vi ".NET Process Tester.vi"() -> ()   [LabVIEW 2019]
uses:
  .NET Process/.NET Process.lvclass
panel:
  out "ErrOut":string
  out "StdOut":string
  in  "Send":bool
  in  "Cmd In":string
  in  "Stop":bool
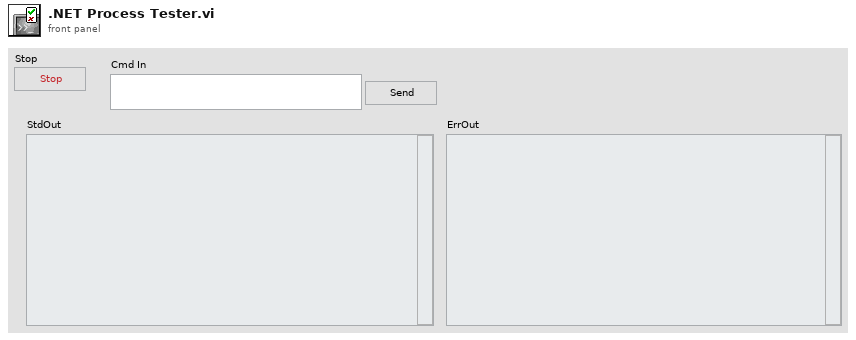
[diagram p1: front panel]
types:
  T1 = cluster{"StdOut Event":refnum<user-event>, "StdErr Event":refnum<user-event>}
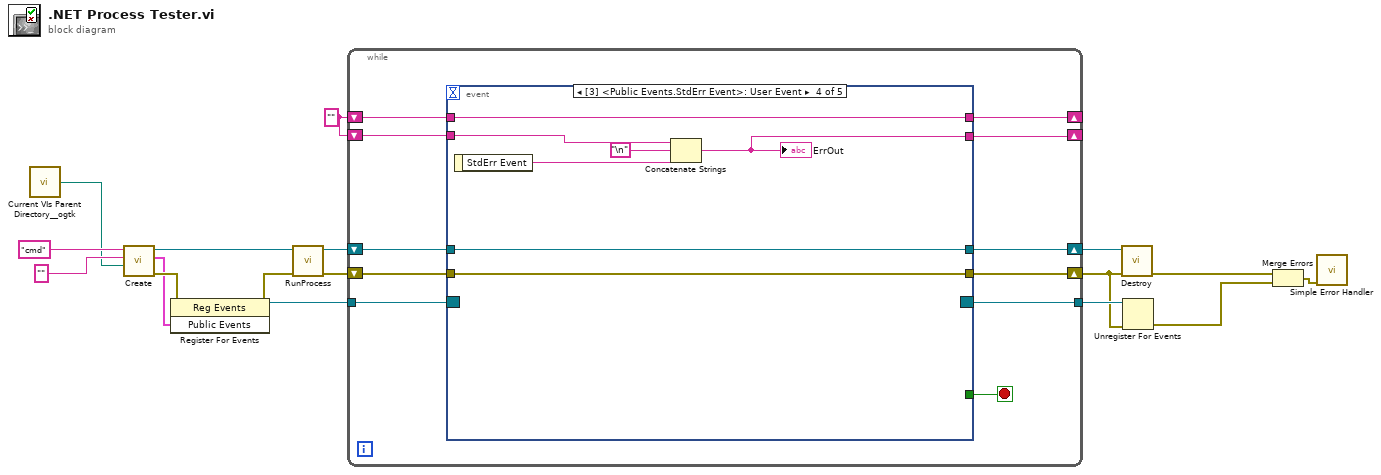
[diagram p0: block diagram]
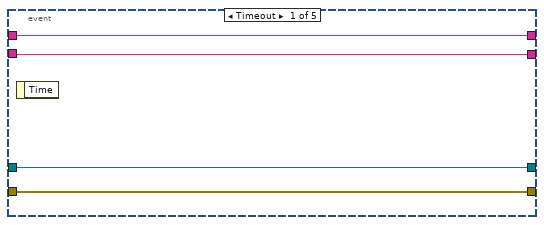
[diagram p2: hidden frame]
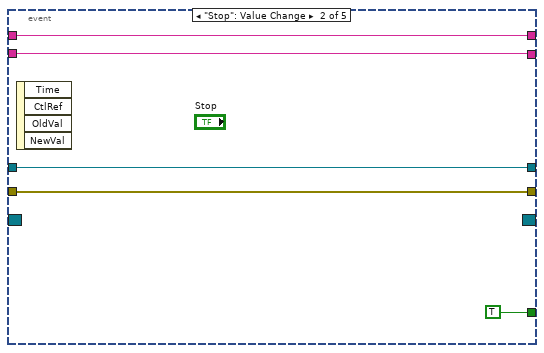
[diagram p3: hidden frame]
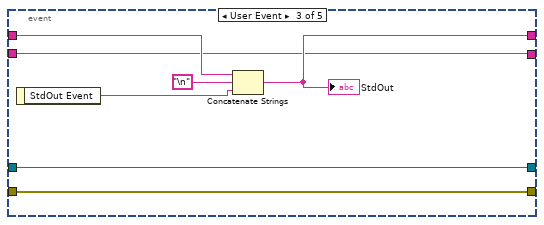
[diagram p4: hidden frame]
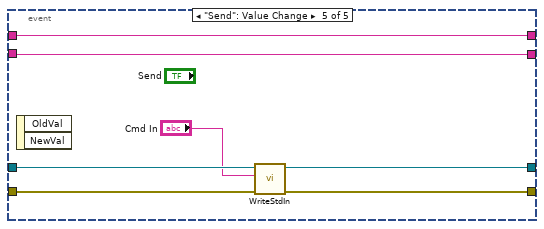
[diagram p5: hidden frame]
diagram:
  w7 = ""
  n1 = call "Current VIs Parent Directory__ogtk.vi"() -> ("Parent Directory (+ Relative)"=w5:path)  [unwired: 5 in]
  n2 = call "Create.vi"("Working Directory (App Directory)"=w5, "Arguments (empty)"="" ("Process File Name"), "Process File Name"="cmd") -> ("error out"=w3:errorcluster, "Public Events"=w1:T1, ".NET Process out"=w15:refnum<class ".NET Process.lvclass">)  [unwired: 6 in]
  n3 = register-events(error in=w3, w1) -> (reference out=w14:refnum<event-registration>, error out=w2:errorcluster)  [unwired: 1 in]
  n4 = call "RunProcess.vi"("error in (no error)"=w2, ".NET Process in"=w15) -> ("error out"=w4:errorcluster, ".NET Process out"=w17:refnum<class ".NET Process.lvclass">)  [unwired: 8 in]
  n5 = while {
    shift-right: [w28] -> w16
    shift-left: w17 -> [w27]
    shift-right: [w25] -> w12
    shift-left: w4 -> [w26]
    tunnel: w14 -> [w24]
    tunnel: [w23] -> w13
    shift-right: [w21] -> _
    shift-left: w7 -> [w22]
    shift-right: [w18] -> _
    shift-left: w7 -> [w19]
    stop <- w20 stop-if-true
    n6 = event shown="[3] <Public Events.StdErr Event>: User Event" {
      selector: w24 -> [_ _ _ _ _]
      dyn-events: [_ _ _ _ _] -> w23
      timeout: _ -> [_ _ _ _ _]
      tunnel: [w32 w37 w44 w51 w58] -> w28
      tunnel: w27 -> [w32 w37 w44 w51 w57]
      tunnel: w26 -> [w31 w36 w43 w50 w55]
      tunnel: [w31 w36 w43 w50 w56] -> w25
      tunnel: w22 -> [w30 w34 w40 w46 w53]
      tunnel: [w30 w34 w41 w46 w53] -> w21
      tunnel: [_ TRUE _ _ _] -> w20
      tunnel: w19 -> [w29 w33 w38 w47 w52]
      tunnel: [w29 w33 w38 w45 w52] -> w18
      event Timeout {
        n7 = event-data() -> ()  [unwired: 1 in, 1 out]
      }
      event "Stop": Value Change {
        n8 = event-data() -> ()  [unwired: 1 in, 4 out]
      }
      event User Event {
        n9 = event-data() -> ("StdOut Event"=w39:string)  [unwired: 1 in]
        n10 = Concatenate Strings(w40, "\n", w39) -> (w41:string)
        "StdOut" <- w41
      }
      event User Event {
        n11 = event-data() -> ("StdErr Event"=w48:string)  [unwired: 1 in]
        n12 = Concatenate Strings(w47, "\n", w48) -> (w45:string)
        "ErrOut" <- w45
      }
      event "Send": Value Change {
        n13 = event-data() -> ()  [unwired: 1 in, 2 out]
        n14 = call-dynamic "WriteStdIn.vi"("error in (no error)"=w55, "Input"="Cmd In", ".NET Process in"=w57) -> ("error out"=w56:errorcluster, ".NET Process out"=w58:refnum<class ".NET Process.lvclass">)  [unwired: 7 in]
      }
    }
  }
  n15 = call-dynamic "Destroy.vi"("error in (no error)"=w12, ".NET Process in"=w16) -> ("error out"=w11:errorcluster)  [unwired: 8 in, 1 out]
  n16 = Unregister For Events(event registration refnum=w13, error in=w12) -> (error out=w10:errorcluster)
  n17 = Merge Errors(w11, w10) -> (w9:errorcluster)
  n18 = call <vilib>:"Simple Error Handler.vi"("error in (no error)"=w9) -> ()  [unwired: 4 in, 5 out]
